vi "Test Comm.vi"() -> ()   [LabVIEW 2021]
uses:
  ChannelCommon/typedef/FIFO Config.ctl
  ChannelCommon/ChannelCommon.lvlib
  ChannelRegistrar/typedef/Datatype CAN.ctl
  ChannelRegistrar/ChannelRegistrar.lvlib
  CIFChannels/Typedef/Direction.ctl
  CIFChannels/CIFChannels.lvclass
  CIF_NIChn_FifoCAN.lvclass
panel:
  out "status":string
  out "pass":bool
  out "error out":errorcluster
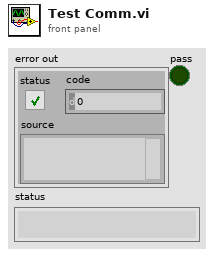
[diagram p1: front panel]
types:
  T1 = typedef "CIFChannels.lvclass/Direction.ctl" = enum16{"Publisher", "Subscriber"}
  T2 = typedef "ChannelCommon.lvlib/FIFO Config.ctl" = cluster{"Depth":u64, "Flags":u64}
  T3 = typedef "ChannelRegistrar.lvlib/Datatype CAN.ctl" = cluster{"payload":u8[], "identifier":u32}
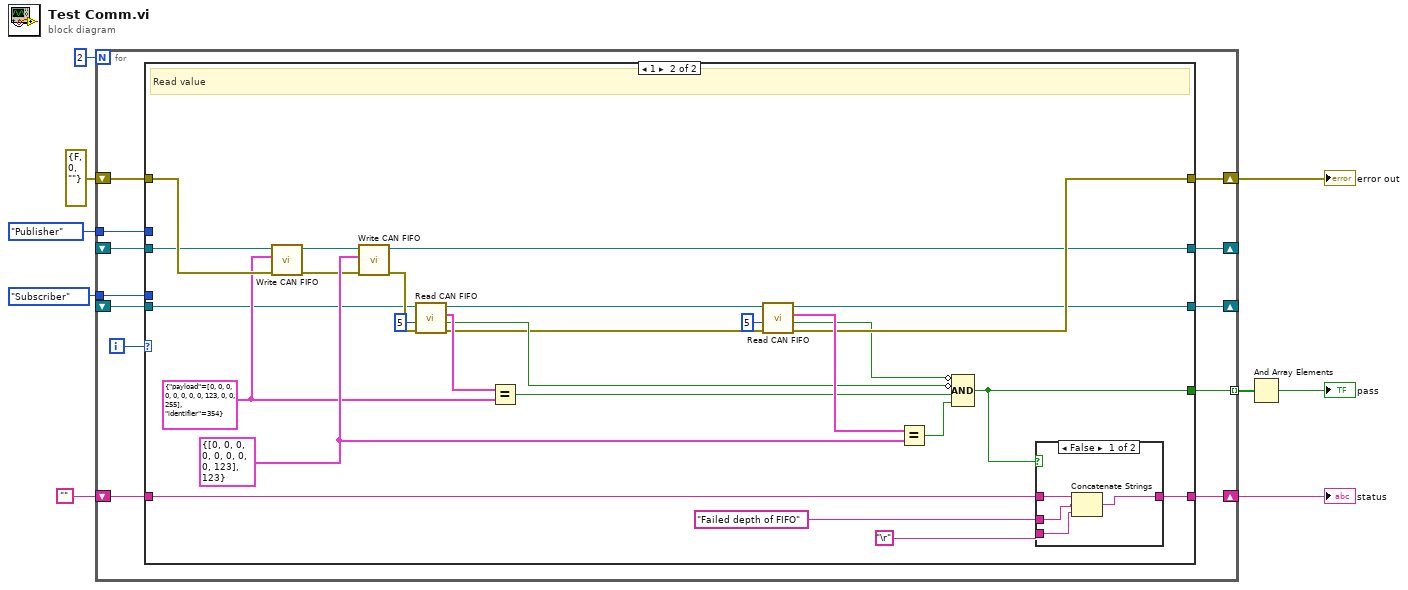
[diagram p0: block diagram]
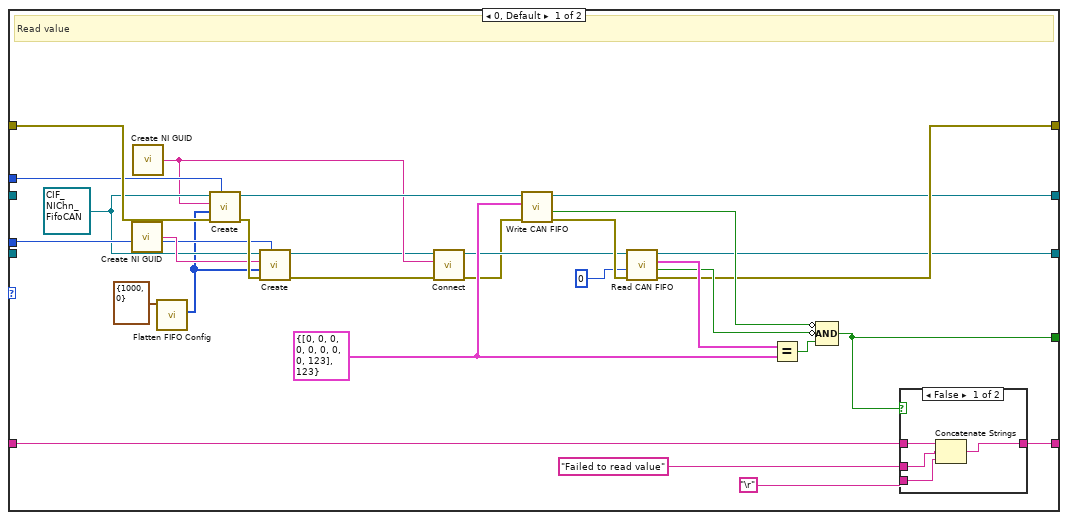
[diagram p2: hidden frame]
diagram:
  n1 = for {
    N: 2 -> [_]
    tunnel: [w21] -> w9 mode=indexing
    shift-right: [w19] -> w4
    shift-left: errorcluster {"status"=FALSE, "code"=0, "source"=""} ("error out") -> [w20]
    shift-right: [w16] -> w5
    shift-left: "" -> [w17]
    tunnel: Direction."Subscriber" ("Direction") -> [w15]
    tunnel: Direction."Publisher" ("Direction") -> [w14]
    shift-right: [w13] -> _
    shift-left: _ -> [w10]
    shift-right: [w12] -> _
    shift-left: _ -> [w11]
    i -> [w18]
    n2 = case shown="1" w18 {
      tunnel: [w45 w76] -> w21
      tunnel: w20 -> [w43 w69]
      tunnel: [w25 w73] -> w19
      tunnel: w17 -> [w50 w80]
      tunnel: [w49 w79] -> w16
      tunnel: w15 -> [w41 _]
      tunnel: w14 -> [w40 _]
      tunnel: [w23 w72] -> w13
      tunnel: [w22 w71] -> w12
      tunnel: w11 -> [_ w56]
      tunnel: w10 -> [_ w57]
      frame 0, Default {
        w34 = T3 {"payload"=[0, 0, 0, 0, 0, 0, 0, 0, 123], "identifier"=123} ("Data")
        w39 = refnum<class "CIF_NIChn_FifoCAN.lvclass"> refnum ("CIF_NIChn_FifoCAN.lvclass")
        # "Read value"
        n3 = call <vilib>:"Create NI GUID.vi"() -> ("NI GUID"=w42:string)
        n4 = call <vilib>:"Create NI GUID.vi"() -> ("NI GUID"=w29:string)
        n5 = call "Flatten FIFO Config.vi"("FIFO Config in"=T2 {"Depth"=1000, "Flags"=0}) -> ("Flattened Data out"=w37:u8[])  [unwired: 8 in, 2 out]
        n6 = call-dynamic "Create.vi"("Direction"=w40, "error in (no error)"=w43, "Custom Config Data"=w37, "Name"=w29, "CIFTag in"=w39) -> ("error out"=w44:errorcluster, "CIFTag out"=w36:refnum<class "CIF_NIChn_FifoCAN.lvclass">)  [unwired: 5 in]
        n7 = call-dynamic "Create.vi"("Direction"=w41, "error in (no error)"=w44, "Custom Config Data"=w37, "Name"=w42, "CIFTag in"=w39) -> ("error out"=w28:errorcluster, "CIFTag out"=w26:refnum<class "CIF_NIChn_FifoCAN.lvclass">)  [unwired: 5 in]
        n8 = call-dynamic "Connect.vi"("error in (no error)"=w28, "Connection Name"=w29, "CIFTag in"=w26) -> ("error out"=w27:errorcluster, "CIFTag out"=w30:refnum<class "CIF_NIChn_FifoCAN.lvclass">)  [unwired: 7 in]
        n9 = call-dynamic "Write CAN FIFO.vi"("error in (no error)"=w27, "Data"=w34, "CIFTag in"=w36) -> ("error out"=w35:errorcluster, "timed out?"=w32:bool, "CIFTag out"=w22:refnum<class "CIF_NIChn_FifoCAN.lvclass">)  [unwired: 6 in]
        n10 = call-dynamic "Read CAN FIFO.vi"("error in (no error)"=w35, "Timeout (ms)"=0, "CIFTag in"=w30) -> ("error out"=w25:errorcluster, "timed out?"=w31:bool, "Data"=w33:T3, "CIFTag out"=w23:refnum<class "CIF_NIChn_FifoCAN.lvclass">)  [unwired: 4 in, 1 out]
        n11 = Equal?(x=w33, y=w34) -> (x = y?=w46:bool)
        n12 = Compound Arithmetic op=AND(invert w32, invert w31, w46) -> (w45:bool)
        n13 = case shown="False" w45 {
          tunnel: w50 -> [w54 w55]
          tunnel: [w51 w55] -> w49
          tunnel: "Failed to read value" -> [w53 _]
          tunnel: "\r" -> [w52 _]
          frame False {
            n14 = Concatenate Strings(w54, w53, w52) -> (w51:string)
          }
          frame True {
          }
        }
      }
      frame 1 {
        w67 = T3 {"payload"=[0, 0, 0, 0, 0, 0, 0, 0, 123, 0, 0, 255], "identifier"=354} ("Data")
        w75 = T3 {"payload"=[0, 0, 0, 0, 0, 0, 0, 0, 123], "identifier"=123} ("Data")
        # "Read value"
        n15 = call-dynamic "Write CAN FIFO.vi"("error in (no error)"=w69, "Data"=w67, "CIFTag in"=w56) -> ("error out"=w62:errorcluster, "CIFTag out"=w70:refnum<class "CIF_NIChn_FifoCAN.lvclass">)  [unwired: 6 in, 1 out]
        n16 = call-dynamic "Write CAN FIFO.vi"("error in (no error)"=w62, "Data"=w75, "CIFTag in"=w70) -> ("CIFTag out"=w71:refnum<class "CIF_NIChn_FifoCAN.lvclass">)  [unwired: 6 in, 2 out]
        n17 = call-dynamic "Read CAN FIFO.vi"("error in (no error)"=w62, "Timeout (ms)"=5, "CIFTag in"=w57) -> ("error out"=w61:errorcluster, "timed out?"=w63:bool, "Data"=w68:T3, "CIFTag out"=w60:refnum<class "CIF_NIChn_FifoCAN.lvclass">)  [unwired: 4 in, 1 out]
        n18 = Equal?(x=w68, y=w67) -> (x = y?=w65:bool)
        n19 = call-dynamic "Read CAN FIFO.vi"("error in (no error)"=w61, "Timeout (ms)"=5, "CIFTag in"=w60) -> ("error out"=w73:errorcluster, "timed out?"=w64:bool, "Data"=w74:T3, "CIFTag out"=w72:refnum<class "CIF_NIChn_FifoCAN.lvclass">)  [unwired: 4 in, 1 out]
        n20 = Equal?(x=w74, y=w75) -> (x = y?=w66:bool)
        n21 = Compound Arithmetic op=AND(invert w64, invert w63, w65, w66) -> (w76:bool)
        n22 = case shown="False" w76 {
          tunnel: w80 -> [w84 w85]
          tunnel: [w81 w85] -> w79
          tunnel: "Failed depth of FIFO" -> [w83 _]
          tunnel: "\r" -> [w82 _]
          frame False {
            n23 = Concatenate Strings(w84, w83, w82) -> (w81:string)
          }
          frame True {
          }
        }
      }
    }
  }
  "error out" <- w4
  "status" <- w5
  n24 = And Array Elements(Boolean array=w9) -> (logical AND=→"pass":bool)
